vi "New.vi"(8 "Error In":errorcluster, 10 "Paths":cluster{"Key":string, "Value":path}[](array[cluster]), 11 "Strings":cluster{"Key":string, "Value":string}[](array[cluster])) -> (0 "Error Out":errorcluster, 3 "Data":refnum<class "Data.lvclass">)   [LabVIEW 2018, in "Toolkit.lvlib" / "Loaders.lvlib" / "Data.lvclass"]
doc: "Creates a new <B>Data</B> partial loader object.\n\n<B>Strings</B> - Key-value clusters where the values are strings of partial Mustache templates stored in memory.\n\n<B>Paths</B> - Key-value clusters where the values are paths to partial Mustache templates stored in a file on disk.\n\n<B>Data</B> - Represents a partial loader implementation capable of loading a partial Mustache template either from memory or in a file based on a value's data type."
uses:
  Data.lvclass
  Data.lvclass/Data.ctl
  Data/String/String.lvclass
  D:/Users/cfield/Code/Field R&D Services/Labstache/src/Toolkit/Data/Datum/Datum.lvclass
  Data/Path/Path.lvclass
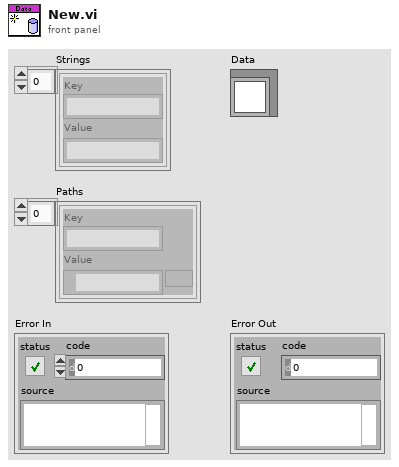
[diagram p1: front panel]
types:
  T1 = cluster{"Key":string, "String":refnum<class "String.lvclass">}
  T2 = cluster{"Key":string, "Path":refnum<class "Path.lvclass">}
  T3 = cluster{"Key":string, "Path":refnum<class "Datum.lvclass">}[]
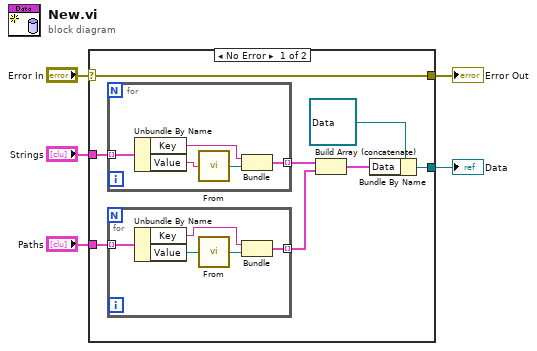
[diagram p0: block diagram]
diagram:
  n1 = case shown="No Error" "Error In" {
    selector: "Error In" -> [w11 w24]
    tunnel: [w12 _] -> w5
    tunnel: [w11 w24] -> w3
    tunnel: "Strings" -> [w10 _]
    tunnel: "Paths" -> [w9 _]
    frame No Error {
      n2 = for {
        tunnel: w10 -> [w23] mode=indexing
        tunnel: [w19] -> w8 mode=indexing
        n3 = Unbundle By Name(w23) -> ("Key"=w21:string, "Value"=w22:string)
        n4 = call "From.vi"("Value"=w22) -> ("String"=w20:refnum<class "String.lvclass">)
        n5 = Bundle("Key"=w21, "String"=w20) -> (w19:T1)  [unwired: 1 in]
      }
      n6 = for {
        tunnel: w9 -> [w18] mode=indexing
        tunnel: [w16] -> w7 mode=indexing
        n7 = Unbundle By Name(w18) -> ("Key"=w17:string, "Value"=w15:path)
        n8 = call "From.vi"("Value"=w15) -> ("Path"=w14:refnum<class "Path.lvclass">)
        n9 = Bundle("Key"=w17, "Path"=w14) -> (w16:T2)  [unwired: 1 in]
      }
      n10 = Build Array (concatenate)(w8, w7) -> (w6:T3)
      n11 = Bundle By Name(cluster=refnum<class "Data.lvclass"> refnum ("Toolkit.lvlib:Loaders.lvlib:Data.lvclass"), "Data"=w6) -> (w12:refnum<class "Data.lvclass">)
    }
    frame Error {
    }
  }
  "Data" <- w5
  "Error Out" <- w3
